vi "Run.vi"(8 "error in (no error)":errorcluster, 11 "Car Wash Console in":refnum<class "Car Wash Display.lvclass">) -> (0 "error out":errorcluster, 3 "Car Wash Console out":refnum<class "Car Wash Display.lvclass">)   [LabVIEW 2016, in "CLD Exam - Car Wash.lvlib" / "Car Wash Display.lvclass"]
doc: "--\nCopyright © 2017 Composed SystemsI All rights reserved.\n\nAuthor: Jon McBee <jon.mcbee@composed.io>\n\nThis library is provided \"AS IS\" ,WITHOUT WARRANTIES OR\nCONDITIONS OF ANY KIND, either express or implied.\n\nComposed Systems -- composed.io\n\nStream 0.0.1.1\nJon McBee - Composed Systems\nCopyright (c) 2017, Composed Systems"
uses:
  Car Wash Display.lvclass
  D:/Repos/Stream/software/Mediator/Classes/Mediated Actor/Mediated Actor.lvclass
  Mediator/Classes/Message Interface/Message Interface.lvclass
  Car Wash Display.lvclass/Car Wash Display.ctl
  Car Wash Option Started Event/Car Wash Option Started.lvclass
  Mediator/Classes/Mediated Actor/Mediated Actor.lvclass
panel:
  out "Elapsed Time (sec)":dbl format="%<%H:%M:%S%1u>t"
  out "Vehicle Out of Position":bool
  out "Air Dry":bool
  out "Tire Shine Foam":bool
  out "Spot Free Rinse":bool
  out "Low Pressure Wax":bool
  out "High Pressure Wash":bool
  out "Pre-Soak":bool
  out "Bug Remover":bool
  out "Wash Entry":string
  out "Under Body Wash":bool
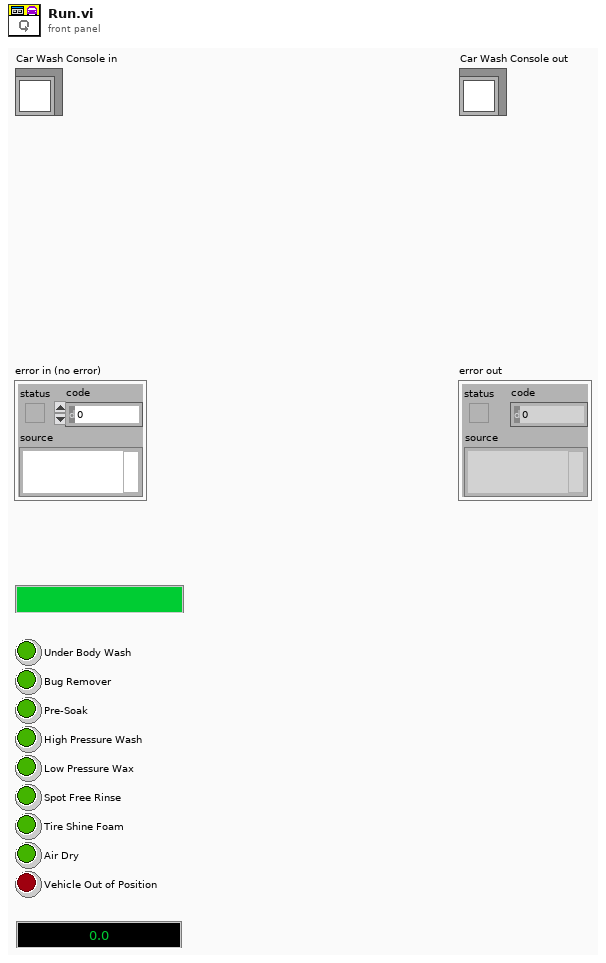
[diagram p1: front panel]
types:
  T1 = cluster{"System Exit":refnum<event-registration>, "To Self":refnum<event-registration>, "Car Wash Started":refnum<event-registration>, "Car Wash Option Started":refnum<event-registration>, "Car Wash Option Finished":refnum<event-registration>, "Car Wash Finished":refnum<event-registration>, "Vehicle Out of Position":refnum<event-registration>}
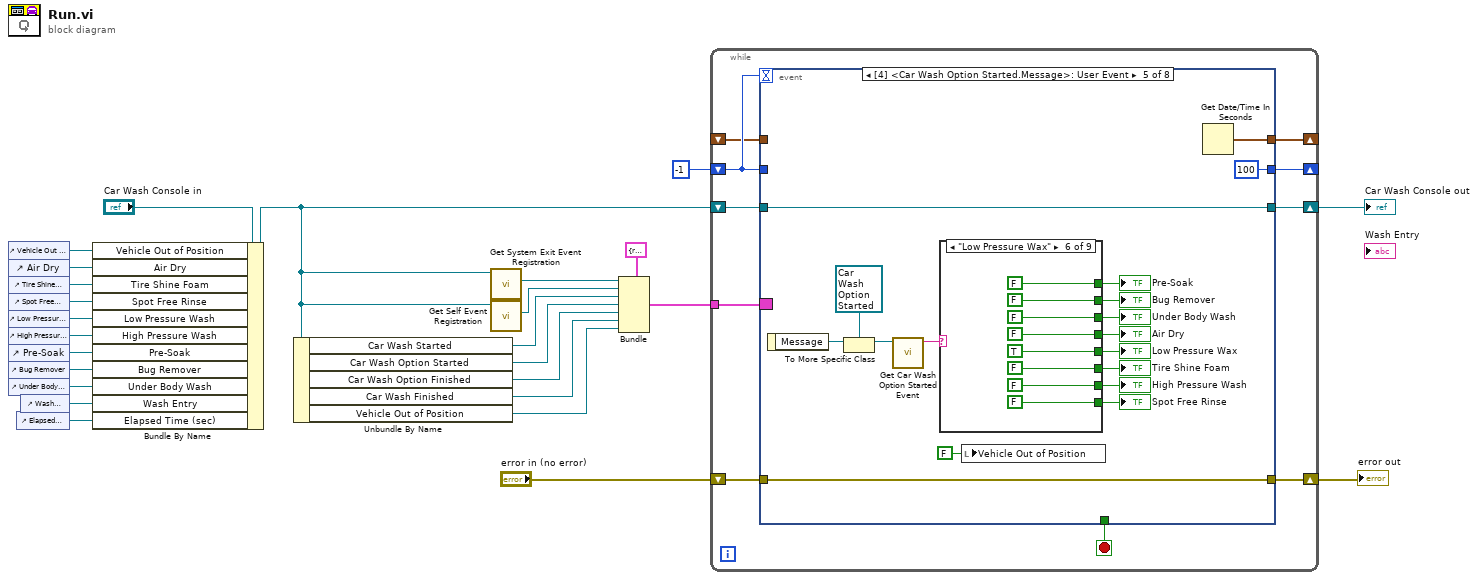
[diagram p0: block diagram]
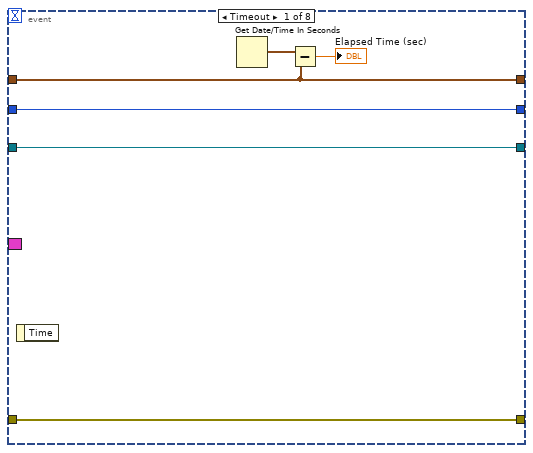
[diagram p2: hidden frame]
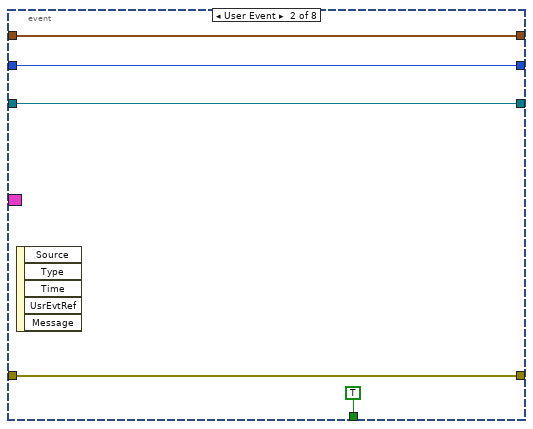
[diagram p3: hidden frame]
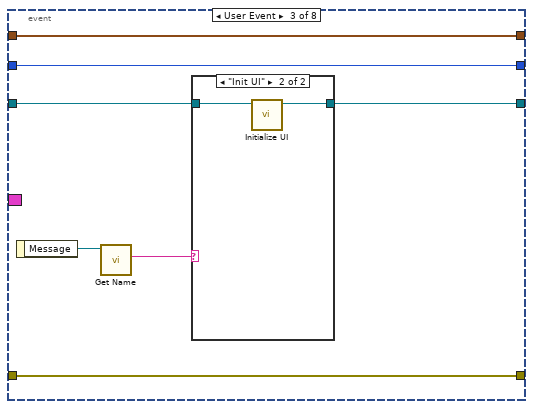
[diagram p4: hidden frame]
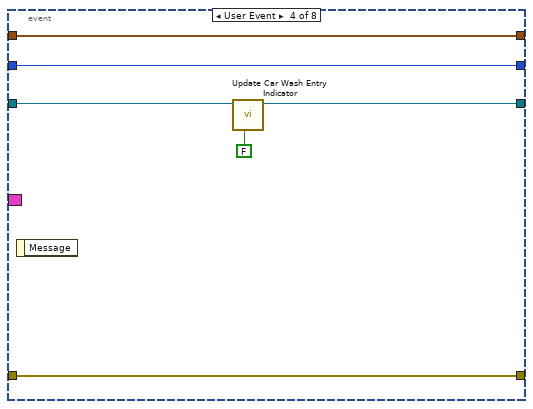
[diagram p6: hidden frame]
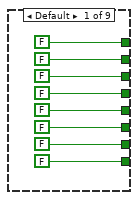
[diagram p7: hidden frame]
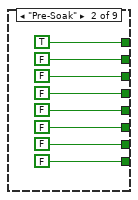
[diagram p8: hidden frame]
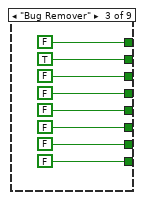
[diagram p9: hidden frame]
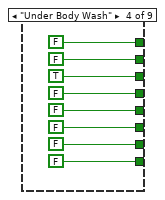
[diagram p10: hidden frame]
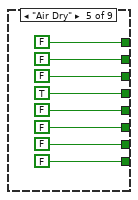
[diagram p11: hidden frame]
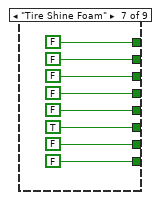
[diagram p12: hidden frame]
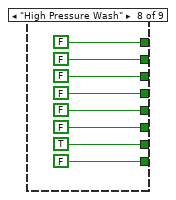
[diagram p13: hidden frame]
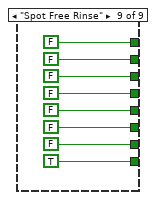
[diagram p14: hidden frame]
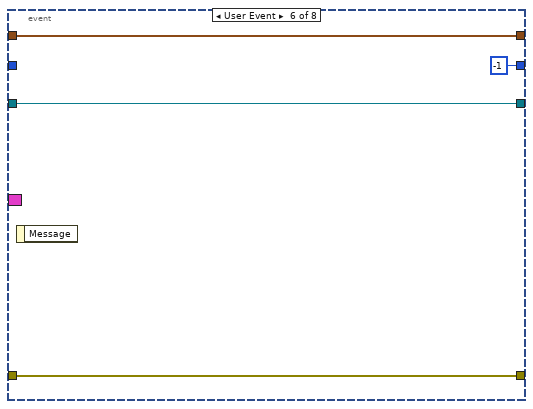
[diagram p15: hidden frame]
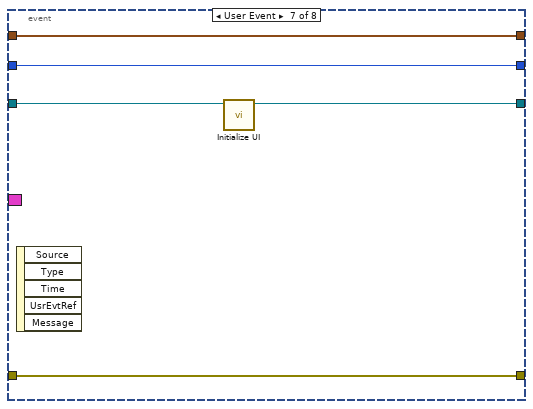
[diagram p16: hidden frame]
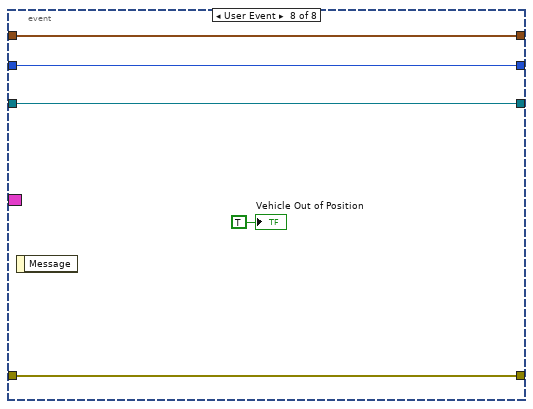
[diagram p17: hidden frame]
diagram:
  n1 = control-ref of="Vehicle Out of Position"() -> (w23:refnum<vi>)
  n2 = control-ref of="Air Dry"() -> (w22:refnum<vi>)
  n3 = control-ref of="Tire Shine Foam"() -> (w21:refnum<vi>)
  n4 = control-ref of="Spot Free Rinse"() -> (w20:refnum<vi>)
  n5 = control-ref of="Low Pressure Wax"() -> (w19:refnum<vi>)
  n6 = control-ref of="High Pressure Wash"() -> (w18:refnum<vi>)
  n7 = control-ref of="Pre-Soak"() -> (w17:refnum<vi>)
  n8 = control-ref of="Bug Remover"() -> (w16:refnum<vi>)
  n9 = control-ref of="Under Body Wash"() -> (w15:refnum<vi>)
  n10 = control-ref of="Elapsed Time (sec)"() -> (w13:refnum<vi>)
  n11 = control-ref of="Wash Entry"() -> (w14:refnum<vi>)
  n12 = Bundle By Name(cluster="Car Wash Console in", "Vehicle Out of Position"=w23, "Air Dry"=w22, "Tire Shine Foam"=w21, "Spot Free Rinse"=w20, "Low Pressure Wash"=w19, "High Pressure Wash"=w18, "Pre-Soak"=w17, "Bug Remover"=w16, "Under Body Wash"=w15, "Wash Entry"=w14, "Elapsed Time (sec)"=w13) -> (w8:refnum<class "Car Wash Display.lvclass">)
  n13 = Unbundle By Name(w8) -> ("Car Wash Started"=w6:refnum<event-registration>, "Car Wash Option Started"=w5:refnum<event-registration>, "Car Wash Option Finished"=w4:refnum<event-registration>, "Car Wash Finished"=w3:refnum<event-registration>, "Vehicle Out of Position"=w1:refnum<event-registration>)
  n14 = call "Get System Exit Event Registration.vi"("Mediated Actor in"=w8) -> ("System Exit Registration"=w11:refnum<event-registration>)  [unwired: 9 in, 1 out]
  n15 = call "Get Self Event Registration.vi"("Mediated Actor in"=w8) -> ("Event Registration Refnum"=w10:refnum<event-registration>)  [unwired: 9 in, 1 out]
  n16 = Bundle(cluster=T1 {"System Exit"=refnum, "To Self"=refnum, "Car Wash Started"=refnum, "Car Wash Option Started"=refnum, "Car Wash Option Finished"=refnum, "Car Wash Finished"=refnum, "Vehicle Out of Position"=refnum} ("output cluster"), "System Exit"=w11, "To Self"=w10, "Car Wash Started"=w6, "Car Wash Option Started"=w5, "Car Wash Option Finished"=w4, "Car Wash Finished"=w3, "Vehicle Out of Position"=w1) -> (w7:T1)
  n17 = while {
    shift-right: [w35] -> w26
    shift-left: w8 -> [w36]
    shift-right: [w33] -> w24
    shift-left: "error in (no error)" -> [w34]
    tunnel: w7 -> [w32]
    shift-right: [w30] -> _
    shift-left: -1 -> [w29]
    shift-right: [w28] -> _
    shift-left: _ -> [w27]
    stop <- w31 stop-if-true
    n18 = event shown="[4] <Car Wash Option Started.Message>: User Event" {
      selector: w32 -> [_ _ _ _ _ _ _ _]
      dyn-events: _ -> [_ _ _ _ _ _ _ _]
      timeout: w29 -> [_ _ _ _ _ _ _ _]
      tunnel: w36 -> [w42 w47 w53 w62 w80 w156 w160 w166]
      tunnel: [w42 w47 w52 w61 w80 w156 w159 w166] -> w35
      tunnel: w34 -> [w41 w46 w54 w63 w79 w155 w161 w165]
      tunnel: [w41 w46 w54 w63 w79 w155 w161 w165] -> w33
      tunnel: [_ TRUE _ _ _ _ _ _] -> w31
      tunnel: [w40 w44 w49 w59 100 -1 w158 w164] -> w30
      tunnel: w29 -> [w40 w44 w49 w59 _ _ w158 w164]
      tunnel: [w38 w43 w48 w58 w65 w153 w157 w163] -> w28
      tunnel: w27 -> [w38 w43 w48 w58 _ w153 w157 w163]
      event Timeout {
        n19 = event-data() -> ()  [unwired: 1 in, 1 out]
        n20 = Get Date/Time In Seconds() -> (seconds since 1Jan1904=w39:timestamp)
        n21 = Subtract(x=w39, y=w38) -> (x-y=→"Elapsed Time (sec)":dbl)
      }
      event User Event {
        n22 = event-data() -> ()  [unwired: 1 in, 5 out]
      }
      event User Event {
        n23 = event-data() -> ("Message"=w51:refnum<class "Message Interface.lvclass">)  [unwired: 1 in]
        n24 = call "Get Name.vi"("Message Interface in"=w51) -> ("Name"=w50:string)  [unwired: 8 in, 2 out]
        n25 = case shown="\"Init UI\"" w50 {
          tunnel: w53 -> [w55 w57]
          tunnel: [w55 w56] -> w52
          frame Default {
          }
          frame "Init UI" {
            n26 = call "Initialize UI.vi"("Car Wash Display in"=w57) -> ("Car Wash Display out"=w56:refnum<class "Car Wash Display.lvclass">)  [unwired: 10 in]
          }
        }
      }
      event User Event {
        n27 = event-data() -> ()  [unwired: 1 in, 1 out]
        n28 = call "Update Car Wash Entry Indicator.vi"("Vacant?"=FALSE, "Car Wash Display in"=w62) -> ("Car Wash Display out"=w61:refnum<class "Car Wash Display.lvclass">)  [unwired: 9 in]
      }
      event User Event {
        n29 = event-data() -> ("Message"=w78:refnum<class "Message Interface.lvclass">)  [unwired: 1 in]
        n30 = To More Specific Class(target class=refnum<class "Car Wash Option Started.lvclass"> refnum ("Car Wash Option Started.lvclass"), reference=w78) -> (specific class reference=w76:refnum<class "Car Wash Option Started.lvclass">)  [unwired: 1 in, 1 out]
        n31 = call "Get Car Wash Option Started Event.vi"("Car Wash Option Started in"=w76) -> ("Option"=w75:string)  [unwired: 9 in, 1 out]
        n32 = case shown="\"Low Pressure Wax\"" w75 {
          tunnel: [FALSE TRUE FALSE FALSE FALSE FALSE FALSE FALSE FALSE] -> w74
          tunnel: [FALSE FALSE TRUE FALSE FALSE FALSE FALSE FALSE FALSE] -> w73
          tunnel: [FALSE FALSE FALSE TRUE FALSE FALSE FALSE FALSE FALSE] -> w72
          tunnel: [FALSE FALSE FALSE FALSE TRUE FALSE FALSE FALSE FALSE] -> w71
          tunnel: [FALSE FALSE FALSE FALSE FALSE TRUE FALSE FALSE FALSE] -> w70
          tunnel: [FALSE FALSE FALSE FALSE FALSE FALSE TRUE FALSE FALSE] -> w69
          tunnel: [FALSE FALSE FALSE FALSE FALSE FALSE FALSE TRUE FALSE] -> w68
          tunnel: [FALSE FALSE FALSE FALSE FALSE FALSE FALSE FALSE TRUE] -> w67
          frame Default {
          }
          frame "Pre-Soak" {
          }
          frame "Bug Remover" {
          }
          frame "Under Body Wash" {
          }
          frame "Air Dry" {
          }
          frame "Low Pressure Wax" {
          }
          frame "Tire Shine Foam" {
          }
          frame "High Pressure Wash" {
          }
          frame "Spot Free Rinse" {
          }
        }
        "Under Body Wash" <- w72
        "Bug Remover" <- w73
        "Pre-Soak" <- w74
        "High Pressure Wash" <- w68
        "Low Pressure Wax" <- w70
        "Spot Free Rinse" <- w67
        "Tire Shine Foam" <- w69
        "Air Dry" <- w71
        n33 = local write "Vehicle Out of Position"(FALSE ("Vehicle Out of Position")) -> ()
        n34 = Get Date/Time In Seconds() -> (seconds since 1Jan1904=w65:timestamp)
      }
      event User Event {
        n35 = event-data() -> ()  [unwired: 1 in, 1 out]
      }
      event User Event {
        n36 = event-data() -> ()  [unwired: 1 in, 5 out]
        n37 = call "Initialize UI.vi"("Car Wash Display in"=w160) -> ("Car Wash Display out"=w159:refnum<class "Car Wash Display.lvclass">)  [unwired: 10 in]
      }
      event User Event {
        n38 = event-data() -> ()  [unwired: 1 in, 1 out]
        "Vehicle Out of Position" <- TRUE ("Vehicle Out of Position")
      }
    }
  }
  "error out" <- w24
  "Car Wash Console out" <- w26
